vi "DB_Info.vi"() -> ()   [LabVIEW 2009]
panel:
  in  "Radio Buttons":enum32{"Use Database", "Radio Selection 2"}(radio)
  in  "password":string="bOsshOg22"
  in  "loginID":string="irm"
  in  "Database":string="irmdb"
  in  "User ID":string
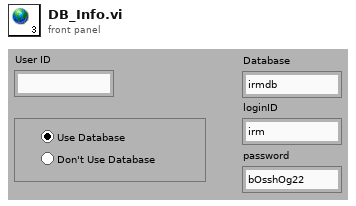
[diagram p1: front panel]
diagram:
